vi "Test_image_display_speed.vi"() -> ()   [LabVIEW 2018]
uses:
  <vilib>/Analysis/baseanly.llb/Unimode.vi
  Tracker.lvlib
  <vilib>/Analysis/NI_AALBase.lvlib
panel:
  out "Histogram Graph 2":T1(graph)
  out "Histogram Graph":T1(graph)
  out "Image Display":T2(plugin-control)
  in  "Colors array input 2":u32[](array[colorbox])=[255, 65535, 6618880, 16776960, 16744448, 16711680]
  out "FPS 2":dbl format="%0.2f"
  in  "Run Button 2":bool
  out "Picture":picture
  in  "Arr. add.":i32=6
  out "FPS":dbl format="%0.2f"
  in  "Image size":i32=660
  in  "Rect color":u32(colorbox)=16777088
  in  "Run Button":bool
  out "Image":T2(plugin-control)
  in  "BGR":u32(colorbox)=8388608
  out "error out":errorcluster
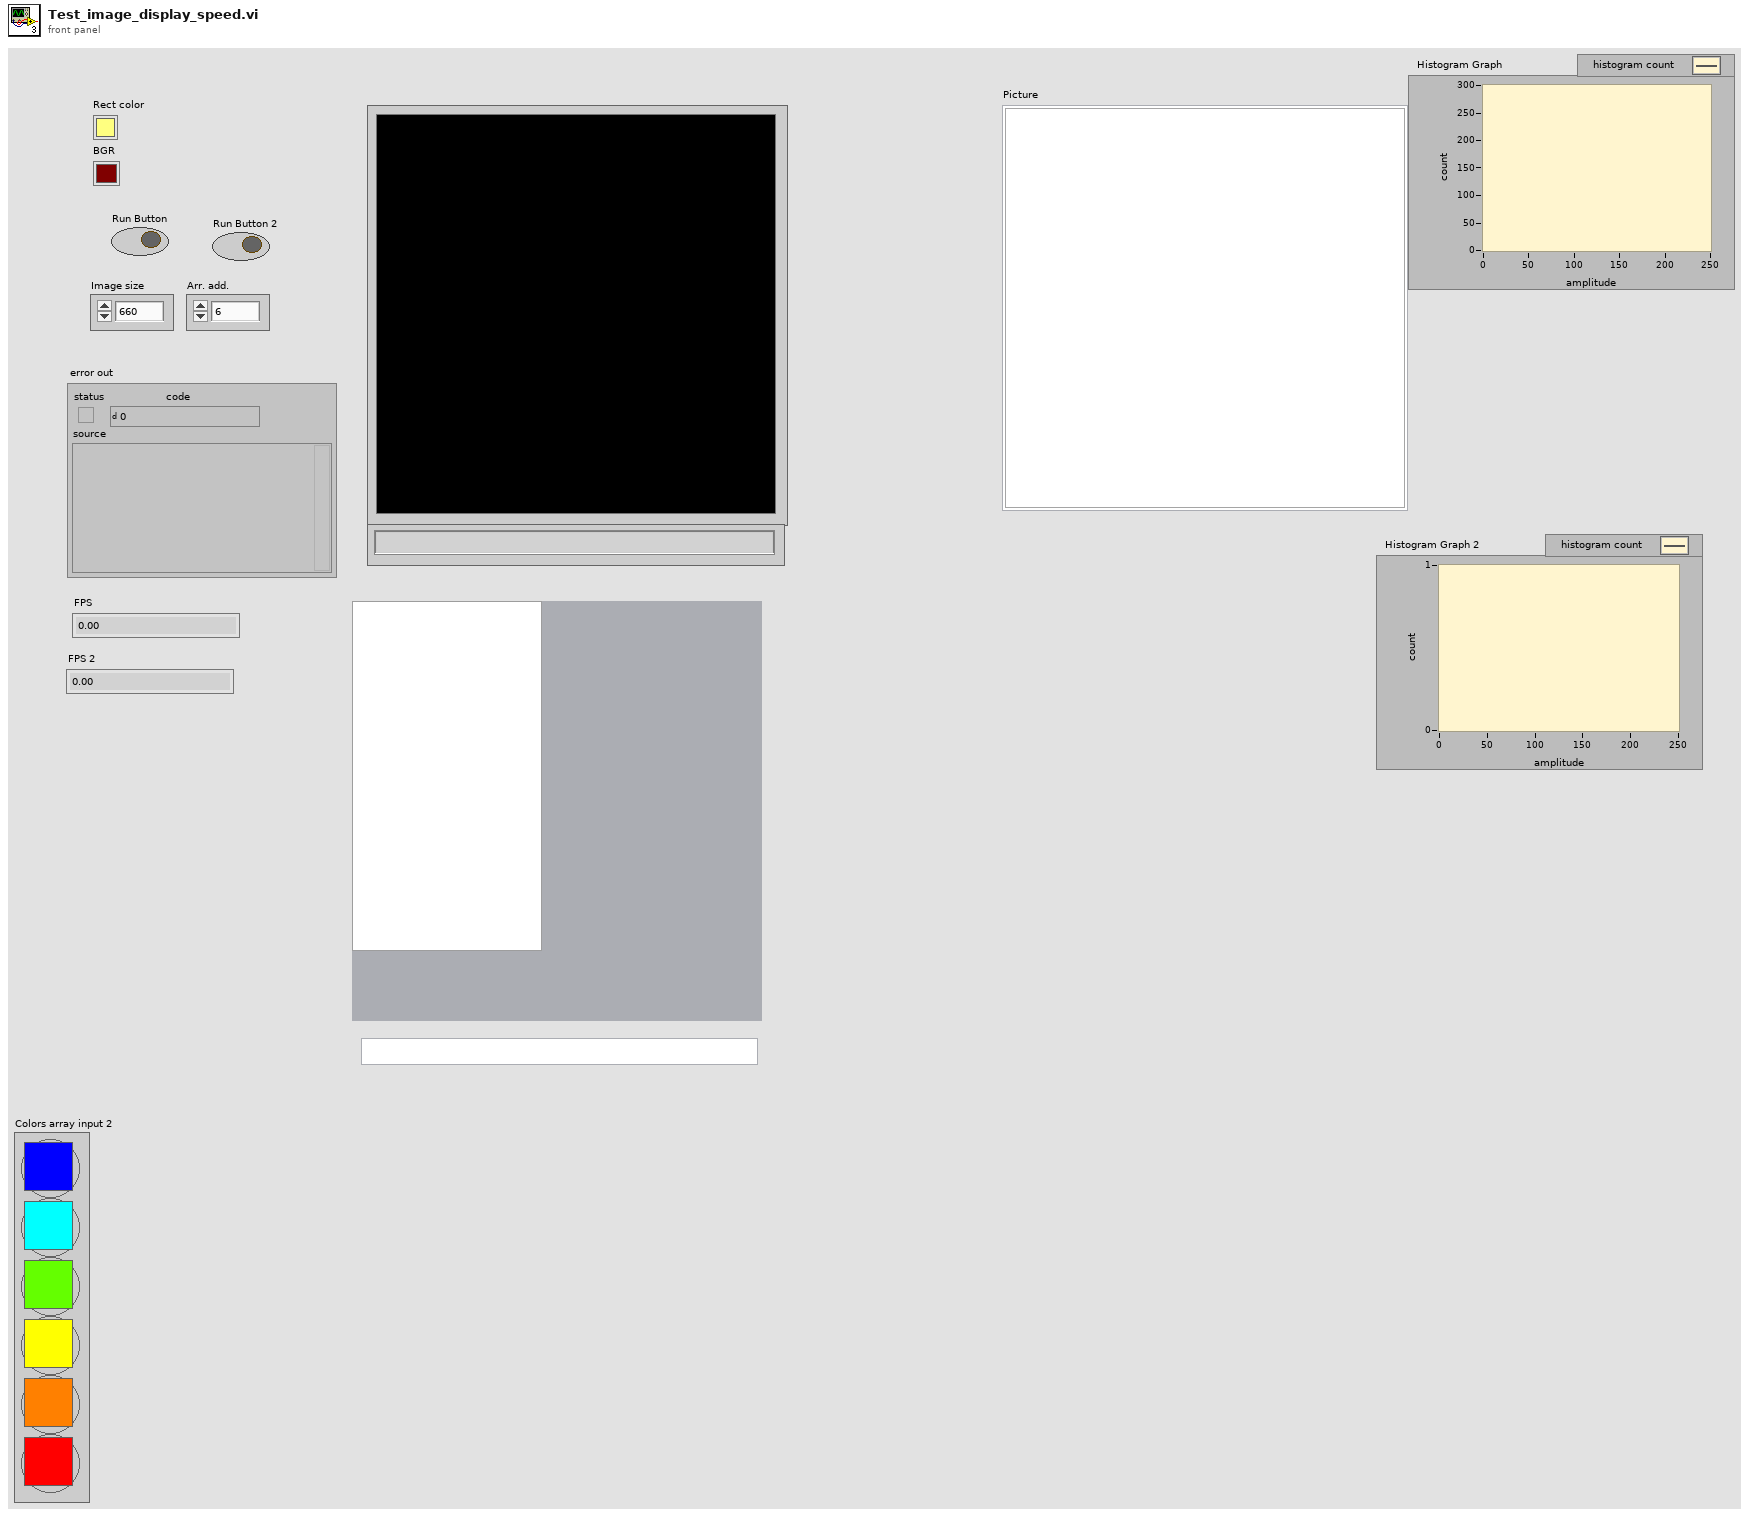
[diagram p1: front panel]
types:
  T1 = cluster{"X Values":dbl[], "Histogram: h(x)":i32[]}
  T2 = typedef "IMAQ Image.ctl" = refnum<image>
  T3 = cluster{"Width":i16, "Style":enum32{"Solid", "Dash", "Dot", "DashDot", "DashDotDot"}}
  T4 = cluster{"Left":i32, "Top":i32, "Right":i32, "Bottom":i32}
  T5 = typedef "Image Type" = u32
  T6 = cluster{"Width":u16, "Style":enum32{"Solid", "Dash", "Dot", "DashDot", "DashDotDot"}}
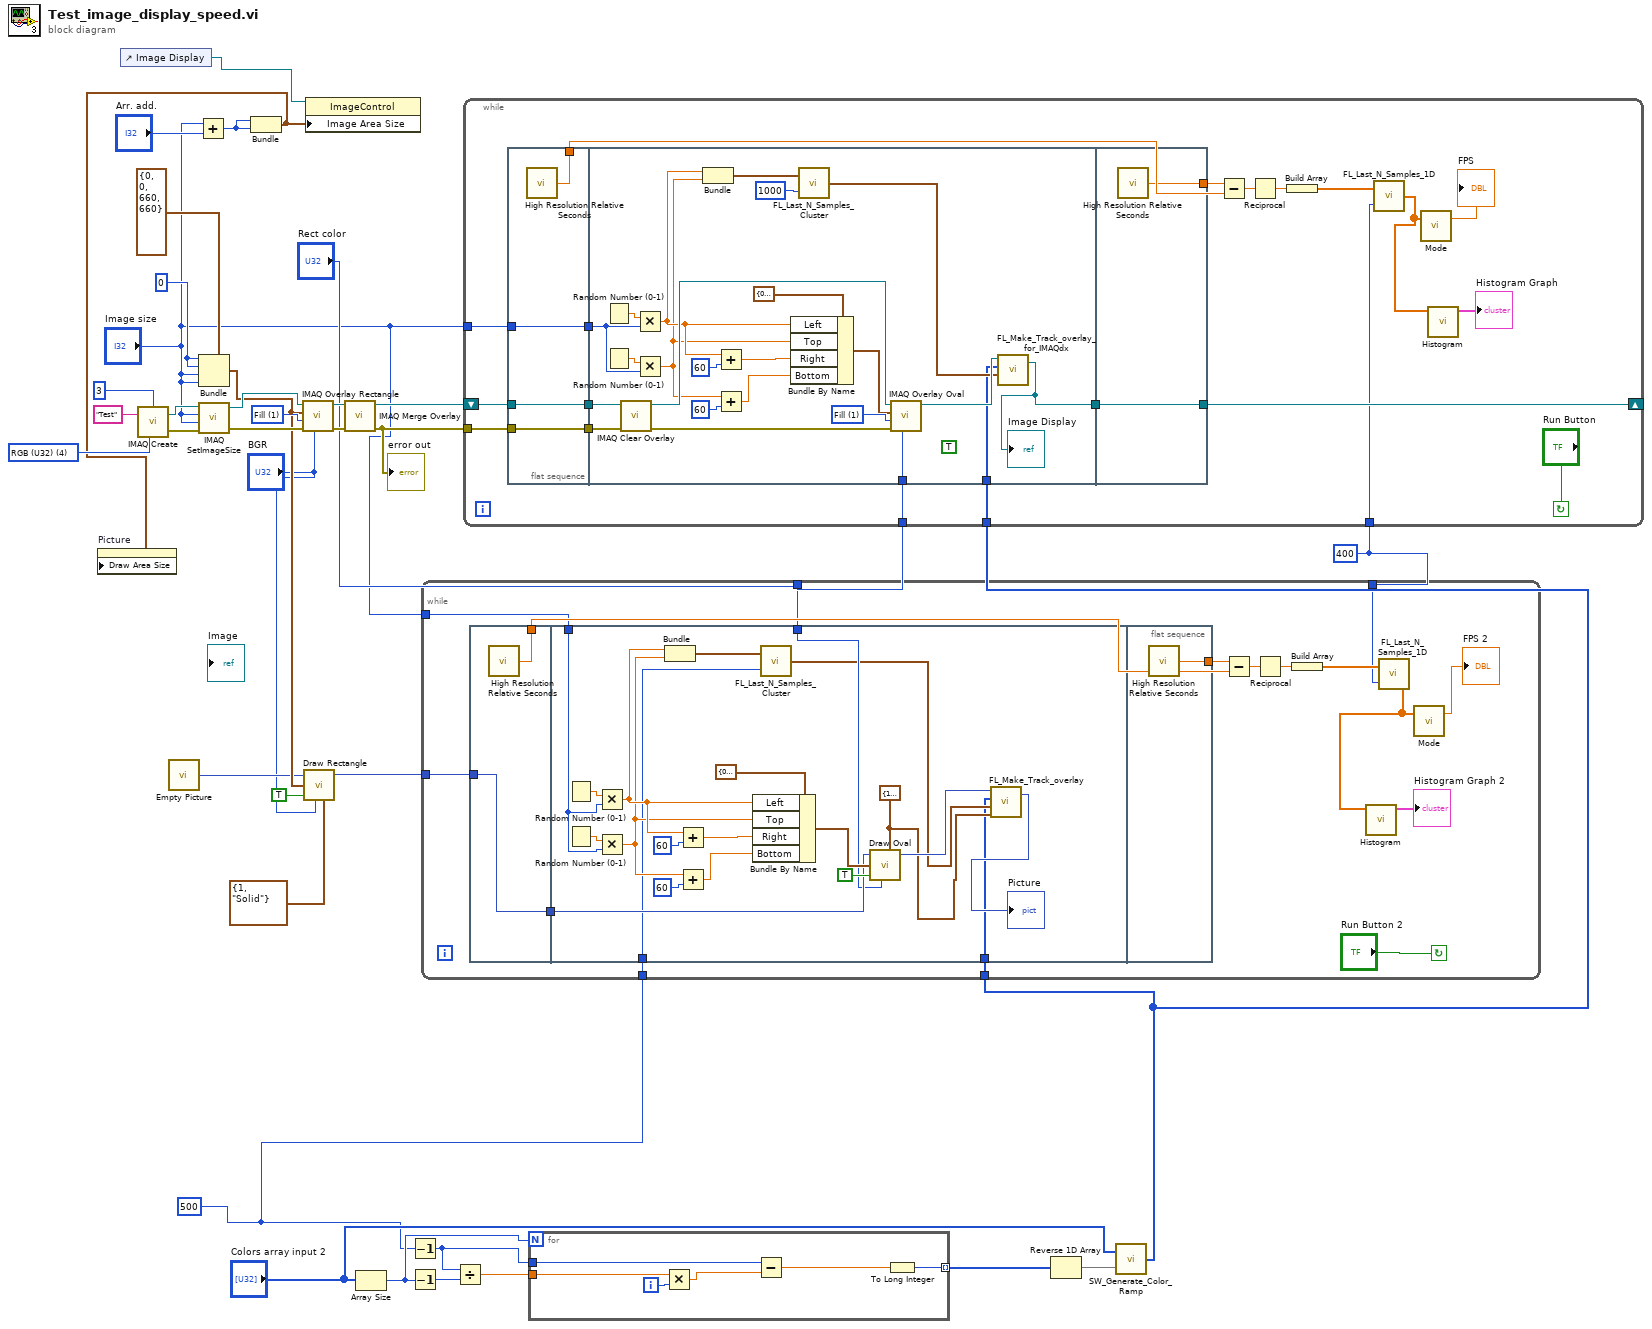
[diagram p0: block diagram]
diagram:
  w3 = u32 400 ("BufferLengthSamples")
  w4 = 500
  w24 = 0 ("Left")
  w27 = u32 1 items=["Frame", "Fill", "Highlight"] ("Drawing Mode (Frame)")
  w32 = T5 4 items=["Grayscale (U8)", "Grayscale (I16)", "Grayscale (SGL)", "Complex (CSG)", "RGB (U32)", "HSL (U32)", "RGB (U64)", "Grayscale (U16)"] ("Image Type")
  n1 = control-ref of="Image Display"() -> (w1:refnum<vi>)
  n2 = call "IMAQ Create"("Border Size"=3, "Image Name"="Test", "Image Type"=w32) -> ("New Image"=w34:T2, "error out"=w33:errorcluster)  [unwired: 2 in]
  n3 = call "Empty Picture"() -> ("empty picture"=w16:picture)
  n4 = Add(x="Image size", y="Arr. add.") -> (x+y=w21:i32)
  n5 = Bundle(cluster=T4 {"Left"=0, "Top"=0, "Right"=660, "Bottom"=660} ("Rectangle"), "Left"=w24, "Top"=w24, "Right"="Image size", "Bottom"="Image size") -> (w20:T4)
  n6 = call "IMAQ SetImageSize"("error in (no error)"=w33, "Y Resolution"="Image size", "X Resolution"="Image size", "Image"=w34) -> ("error out"=w30:errorcluster, "Image Out"=w31:T2)  [unwired: 1 in]
  n7 = Bundle(w21, w21) -> (w18:cluster{i32, i32})  [unwired: 1 in]
  n8 = property on="Picture" class="Pict"("Draw Area Size"=w18) -> ()  [unwired: 2 in, 2 out]
  n9 = call "IMAQ Overlay Rectangle"("Color"="BGR", "error in (no error)"=w30, "Drawing Mode (Frame)"=w27, "Rectangle"=w20, "Image"=w31) -> ("error out"=w28:errorcluster, "Image Out"=w29:T2)  [unwired: 5 in]
  n10 = call <vilib>:"Draw Rectangle.vi"("picture"=w16, "rect"=w20, "fill?(F)"=TRUE, "color(black)"="BGR", "pen"=T3 {"Width"=1, "Style"=enum."Solid"}) -> ("new picture"=w13:picture)  [unwired: 4 in]
  n11 = property class="ImageControl"(reference=w1, "Image Area Size"=w18) -> ()  [unwired: 1 in, 2 out]
  n12 = call "IMAQ Merge Overlay"("error in (no error)"=w28, "Image Src"=w29) -> ("error out"=w23:errorcluster, "Image Dst Out"=w26:T2)  [unwired: 8 in]
  "error out" <- w23
  n13 = Array Size(array="Colors array input 2") -> (size(s)=w6:i32)
  n14 = Decrement(x=w4) -> (x-1=w7:i32)
  n15 = Decrement(x=w6) -> (x-1=w10:i32)
  n16 = Divide(x=w7, y=w10) -> (x/y=w11:dbl)
  n17 = for {
    N: w6 -> [_]
    tunnel: [w37] -> w9 mode=indexing
    tunnel: w7 -> [w42]
    tunnel: w11 -> [w40]
    i -> [w38]
    n18 = Multiply(x=w40, y=w38) -> (x*y=w41:dbl)
    n19 = Subtract(x=w42, y=w41) -> (x-y=w39:dbl)
    n20 = To Long Integer(number=w39) -> (32bit integer=w37:i32)
  }
  n21 = Reverse 1D Array(array=w9) -> (reversed array=w8:i32[])
  n22 = call "SW_Generate_Color_Ramp.vi"("Colors rel. pos."=w8, "Colors array"="Colors array input 2") -> ("Colors array"=w2:u32[])
  n23 = while {
    tunnel: "Rect color" -> [w52]
    tunnel: w13 -> [w50]
    tunnel: "Image size" -> [w49]
    tunnel: w2 -> [w48]
    tunnel: w4 -> [w47]
    tunnel: w3 -> [w46]
    stop <- "Run Button 2" continue-if-true
    n24 = flat-sequence {
      tunnel: [w60] -> w53
      tunnel: [w59] -> w51
      tunnel: w50 -> [w59]
      tunnel: w52 -> [w67]
      tunnel: w51 -> [w69]
      tunnel: w49 -> [w68]
      tunnel: w48 -> [w62]
      tunnel: w47 -> [w61]
      tunnel: [w82] -> w54
      frame #0 {
        n25 = call <vilib>:"High Resolution Relative Seconds.vi"() -> ("relative seconds"=w60:dbl)
      }
      frame #1 {
        w63 = T6 {"Width"=1, "Style"=enum."Solid"} ("pen")
        n26 = Random Number (0-1)() -> (number: 0 to 1=w76:dbl)
        n27 = Random Number (0-1)() -> (number: 0 to 1=w75:dbl)
        n28 = Multiply(x=w76, y=w68) -> (x*y=w74:dbl)
        n29 = Multiply(x=w75, y=w68) -> (x*y=w73:dbl)
        n30 = Bundle(w74, w73) -> (w72:cluster{dbl, dbl})  [unwired: 1 in]
        n31 = Add(x=w74, y=60) -> (x+y=w78:dbl)
        n32 = Add(x=w73, y=60) -> (x+y=w77:dbl)
        n33 = Bundle By Name(cluster=T4 {"Left"=0, "Top"=0, "Right"=0, "Bottom"=0} ("Rectangle"), "Left"=w74, "Top"=w73, "Right"=w78, "Bottom"=w77) -> (w71:T4)
        n34 = call "FL_Last_N_Samples_Cluster.vi"("BufferLengthSamples"=w61, "Input cluster"=w72) -> ("Output 1D array of clusters"=w64:cluster{"X":dbl, "Y":dbl}[])
        n35 = call <vilib>:"Draw Oval.vi"("picture"=w69, "rect"=w71, "fill?(F)"=TRUE, "color(black)"=w67, "pen"=w63) -> ("new picture"=w66:picture)  [unwired: 4 in]
        n36 = call "FL_Make_Track_overlay.vi"("Pen properties"=w63, "Full track array"=w64, "Colors array input"=w62, "Picture in"=w66) -> ("Picture out"=→"Picture":picture)  [unwired: 3 in]
      }
      frame #2 {
        n37 = call <vilib>:"High Resolution Relative Seconds.vi"() -> ("relative seconds"=w82:dbl)
      }
    }
    n38 = Subtract(x=w54, y=w53) -> (x-y=w55:dbl)
    n39 = Reciprocal(x=w55) -> (1/x=w56:dbl)
    n40 = Build Array(w56) -> (w57:dbl[])
    n41 = call "FL_Last_N_Samples_1D.vi"("BufferLengthSamples"=w46, "Input Array"=w57) -> ("Output Array"=w43:dbl[])
    n42 = call <vilib>:"Histogram.vi"("X"=w43) -> ("Histogram Graph"=→"Histogram Graph 2":T1)  [unwired: 7 in, 3 out]
    n43 = call-poly <vilib>:"Mode.vi"("X"=w43) -> ("mode"=→"FPS 2":dbl)  [unwired: 1 in, 1 out]
  }
  n44 = while {
    tunnel: w23 -> [w101]
    shift-right: [w99] -> _
    shift-left: w26 -> [w100]
    tunnel: "Image size" -> [w98]
    tunnel: "Rect color" -> [w88]
    tunnel: w3 -> [w87]
    tunnel: w2 -> [w85]
    stop <- "Run Button" continue-if-true
    n45 = flat-sequence {
      tunnel: w98 -> [w104]
      tunnel: w100 -> [w105]
      tunnel: w101 -> [w106]
      tunnel: [w106] -> w97
      tunnel: [w105] -> w96
      tunnel: [w104] -> w95
      tunnel: [w103] -> w93
      tunnel: w97 -> [w129]
      tunnel: w96 -> [w128]
      tunnel: w95 -> [w117]
      tunnel: [w107] -> w94
      tunnel: w88 -> [w111]
      tunnel: w85 -> [w108]
      tunnel: [w131] -> w99
      tunnel: w94 -> [w131]
      tunnel: [w130] -> w92
      frame #0 {
        n46 = call <vilib>:"High Resolution Relative Seconds.vi"() -> ("relative seconds"=w103:dbl)
      }
      frame #1 {
        (unwired) TRUE ("Maintain Width?")
        w121 = u32 1 items=["Frame", "Fill", "Highlight"] ("Drawing Mode (Frame)")
        n47 = Random Number (0-1)() -> (number: 0 to 1=w119:dbl)
        n48 = Random Number (0-1)() -> (number: 0 to 1=w118:dbl)
        n49 = call "IMAQ Clear Overlay"("error in (no error)"=w129, "Image"=w128) -> ("error out"=w120:errorcluster, "Image Out"=w122:T2)  [unwired: 8 in]
        n50 = Multiply(x=w119, y=w117) -> (x*y=w115:dbl)
        n51 = Multiply(x=w118, y=w117) -> (x*y=w114:dbl)
        n52 = Bundle(w115, w114) -> (w113:cluster{dbl, dbl})  [unwired: 1 in]
        n53 = Add(x=w115, y=60) -> (x+y=w124:dbl)
        n54 = Add(x=w114, y=60) -> (x+y=w123:dbl)
        n55 = Bundle By Name(cluster=T4 {"Left"=0, "Top"=0, "Right"=0, "Bottom"=0} ("Rectangle"), "Left"=w115, "Top"=w114, "Right"=w124, "Bottom"=w123) -> (w116:T4)
        n56 = call "FL_Last_N_Samples_Cluster.vi"("BufferLengthSamples"=u32 1000, "Input cluster"=w113) -> ("Output 1D array of clusters"=w109:cluster{"X":dbl, "Y":dbl}[])
        n57 = call "IMAQ Overlay Oval"("Color"=w111, "error in (no error)"=w120, "Drawing Mode (Frame)"=w121, "Bounding Rectangle"=w116, "Image"=w122) -> ("Image Out"=w110:T2)  [unwired: 5 in, 1 out]
        n58 = call "FL_Make_Track_overlay_for_IMAQdx.vi"("Full track array"=w109, "Colors array input"=w108, "Image In"=w110) -> ("Image Out"=w107:T2)  [unwired: 4 in]
        "Image Display" <- w107
      }
      frame #2 {
        n59 = call <vilib>:"High Resolution Relative Seconds.vi"() -> ("relative seconds"=w130:dbl)
      }
    }
    n60 = Subtract(x=w92, y=w93) -> (x-y=w91:dbl)
    n61 = Reciprocal(x=w91) -> (1/x=w90:dbl)
    n62 = Build Array(w90) -> (w89:dbl[])
    n63 = call "FL_Last_N_Samples_1D.vi"("BufferLengthSamples"=w87, "Input Array"=w89) -> ("Output Array"=w84:dbl[])
    n64 = call-poly <vilib>:"Mode.vi"("X"=w84) -> ("mode"=→"FPS":dbl)  [unwired: 1 in, 1 out]
    n65 = call <vilib>:"Histogram.vi"("X"=w84) -> ("Histogram Graph"=→"Histogram Graph":T1)  [unwired: 7 in, 3 out]
  }
